vi "Read Element of Sections by Name.vi"(8 "error in (no error)":errorcluster, 10 "Section Name":string, 11 "Configuration in":refnum<class "Configuration.lvclass">) -> (0 "error out":errorcluster, 1 "Found?":bool, 2 "Section":refnum<class "Section.lvclass">, 3 "Configuration out":refnum<class "Configuration.lvclass">)   [LabVIEW 2014, in "Configuration.lvlib" / "Configuration.lvclass"]
doc: "Read section by name from class private data."
uses:
  Configuration.lvclass
  Section/Section.lvclass
  Configuration.lvclass/Configuration.ctl
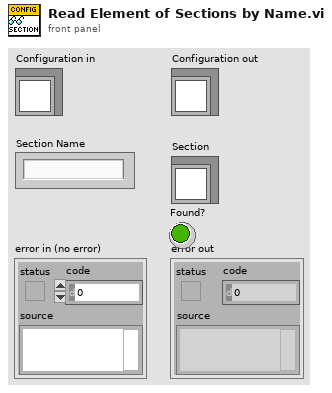
[diagram p1: front panel]
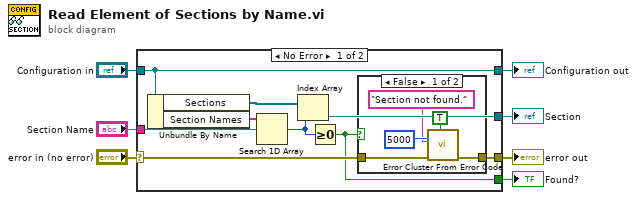
[diagram p0: block diagram]
diagram:
  n1 = case shown="No Error" "error in (no error)" {
    selector: "error in (no error)" -> [w10 w23]
    tunnel: [w8 w23] -> w6
    tunnel: [w16 w24] -> w4
    tunnel: "Configuration in" -> [w16 w24]
    tunnel: [w14 _] -> w3
    tunnel: "Section Name" -> [w12 _]
    tunnel: [w9 _] -> w1
    frame No Error {
      n2 = Unbundle By Name(w16) -> ("Sections"=w15:refnum<class "Section.lvclass">[], "Section Names"=w13:string[])
      n3 = Search 1D Array(1D array=w13, element=w12) -> (index of element=w11:i32)  [unwired: 1 in]
      n4 = Index Array(array=w15, index=w11) -> (element=w14:refnum<class "Section.lvclass">)
      n5 = Greater Or Equal To 0?(x=w11) -> (x >= 0?=w9:bool)
      n6 = case shown="False" w9 {
        tunnel: w10 -> [w18 w22]
        tunnel: [w17 w22] -> w8
        frame False {
          n7 = call <vilib>:"Error Cluster From Error Code.vi"("show call chain? (False)"=TRUE, "error in (no error)"=w18, "error message (\"\")"="Section not found." ("error message (\"\")"), "error code (0)"=5000) -> ("error out"=w17:errorcluster)  [unwired: 5 in]
        }
        frame True {
        }
      }
    }
    frame Error {
    }
  }
  "error out" <- w6
  "Configuration out" <- w4
  "Section" <- w3
  "Found?" <- w1
